vi "property sysdef array tester.vi"() -> ()   [LabVIEW 2019]
uses:
  JSON parsing/propertySysDefPage.ctl
  JSON parsing/EDSjsonStructure.ctl
  JSON parsing/enum.ctl
  JSON parsing/property.ctl
  JSON parsing/command.ctl
  JSON parsing/scale.ctl
  JSON parsing/physicalChannel.ctl
  JSON parsing/register.ctl
panel:
  out "error out":errorcluster
  in  "SLSC EDS module":T1
  out "Properties":T8[](array[typedef])
  # "not working\nregisterMap->registers->initialValue"
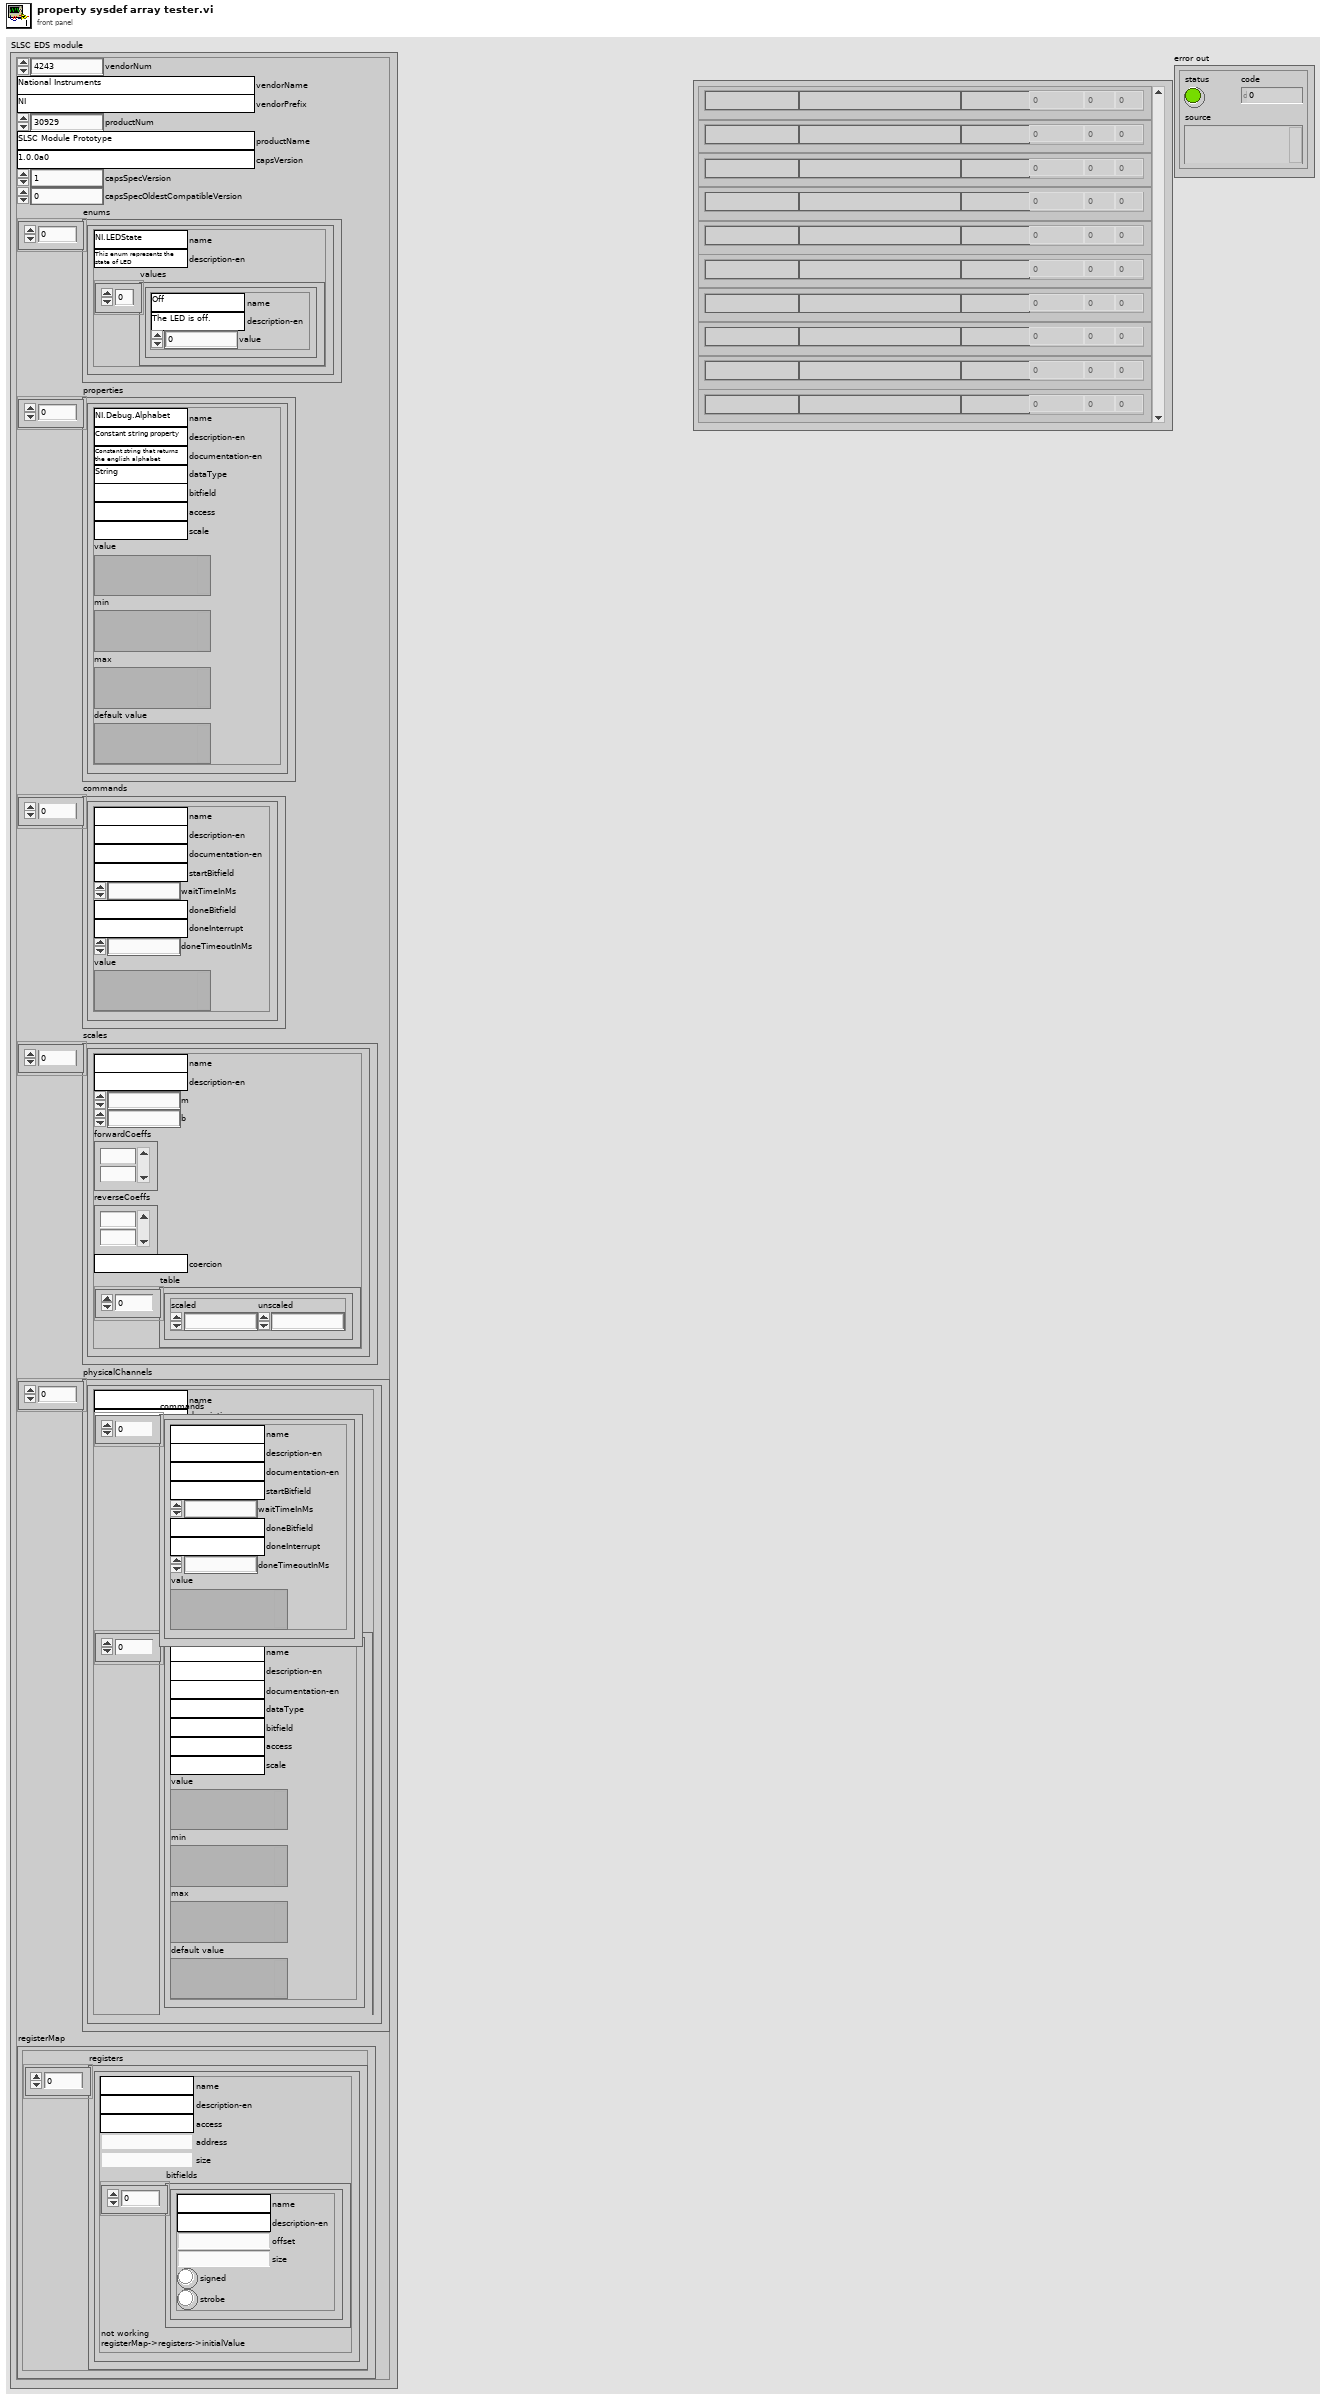
[diagram p1: front panel]
types:
  T1 = typedef "EDSjsonStructure.ctl" = cluster{"vendorNum":u32, "vendorName":string, "vendorPrefix":string, "productNum":u32, "productName":string, "capsVersion":string, "capsSpecVersion":u32, "capsSpecOldestCompatibleVersion":u32, "enums":T2[], "properties":T3[], "commands":T4[], "scales":T5[], "physicalChannels":T6[], "registerMap":cluster{"registers":T7[]}}
  T2 = typedef "enum.ctl" = cluster{"name":string, "description-en":string, "values":cluster{"name":string, "description-en":string, "value":i32}[]}
  T3 = typedef "property.ctl" = cluster{"name":string, "description-en":string, "documentation-en":string, "dataType":string, "bitfield":string, "access":string, "scale":string, "value":variant, "min":variant, "max":variant, "default value":variant}
  T4 = typedef "command.ctl" = cluster{"name":string, "description-en":string, "documentation-en":string, "startBitfield":string, "waitTimeInMs":i32, "doneBitfield":string, "doneInterrupt":string, "doneTimeoutInMs":i32, "value":variant}
  T5 = typedef "scale.ctl" = cluster{"name":string, "description-en":string, "m":dbl, "b":dbl, "forwardCoeffs":dbl[], "reverseCoeffs":dbl[], "coercion":string, "table":cluster{"scaled":dbl, "unscaled":dbl}[]}
  T6 = typedef "physicalChannel.ctl" = cluster{"name":string, "description-en":string, "commands":T4[], "properties":T3[]}
  T7 = typedef "register.ctl" = cluster{"name":string, "description-en":string, "access":string, "address":u32, "size":u32, "bitfields":cluster{"name":string, "description-en":string, "offset":u32, "size":u32, "signed":bool, "strobe":bool}[]}
  T8 = typedef "propertySysDefPage.ctl" = cluster{"name":string, "description-en":string, "dataType":string, "value":dbl, "min":dbl, "max":dbl}
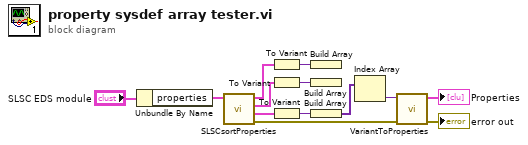
[diagram p0: block diagram]
diagram:
  n1 = Unbundle By Name("SLSC EDS module") -> ("properties"=w5:T3[])
  n2 = call "SLSCsortProperties.vi"("properties"=w5) -> ("Error Out"=w3:errorcluster, "ReadWrite properties"=w8:T3[], "WriteOnly properties"=w9:T3[], "ReadOnly properties"=w12:T3[])  [unwired: 7 in]
  n3 = To Variant(anything=w12) -> (Variant=w13:variant)
  n4 = To Variant(anything=w9) -> (Variant=w11:variant)
  n5 = To Variant(anything=w8) -> (Variant=w10:variant)
  n6 = Build Array(w13) -> ()  [unwired: 1 out]
  n7 = Build Array(w11) -> ()  [unwired: 1 out]
  n8 = Build Array(w10) -> (w4:variant[])
  n9 = Index Array(array=w4) -> (element=w6:variant)  [unwired: 1 in]
  n10 = call "VariantToProperties.vi"("error in (no error)"=w3, "Variant"=w6) -> ("error out"=→"error out":errorcluster, "Properties"=→"Properties":T8[])  [unwired: 8 in]
